vi "PQsyncQueryCommand.vi"(8 "error in (no error)":errorcluster, 9 "query":string, 11 "conn":u64) -> (0 "error out":errorcluster, 1 "PQresultStatus":T1(ring), 2 "PGresult":u64, 3 "conn out":u64, 4 "PQresultErrorMessage":string)   [LabVIEW 2019, in "libpqutility64.lvlib"]
doc: "Synchrounus Communication with PostgreSQL Database.\nSee PostgreSQL c-lib doku for further information."
uses:
  libpqutility64.lvlib
  libpqlv64/libpqlv64.lvlib
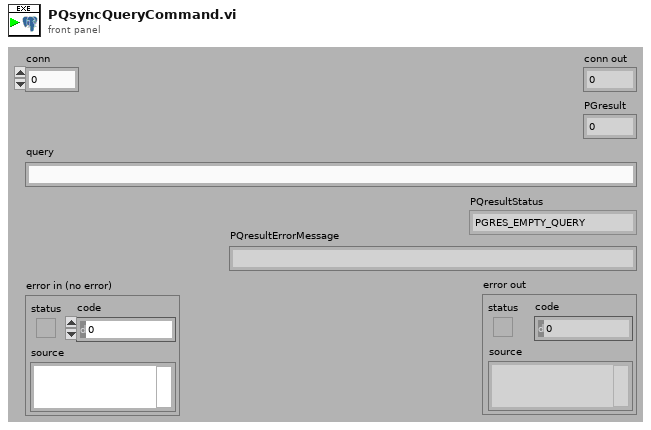
[diagram p1: front panel]
types:
  T1 = enum32{"PGRES_EMPTY_QUERY", "PGRES_COMMAND_OK", "PGRES_TUPLES_OK", "PGRES_COPY_OUT", "PGRES_COPY_IN", "PGRES_BAD_RESPONSE", "PGRES_NONFATAL_ERROR", "PGRES_FATAL_ERROR"}
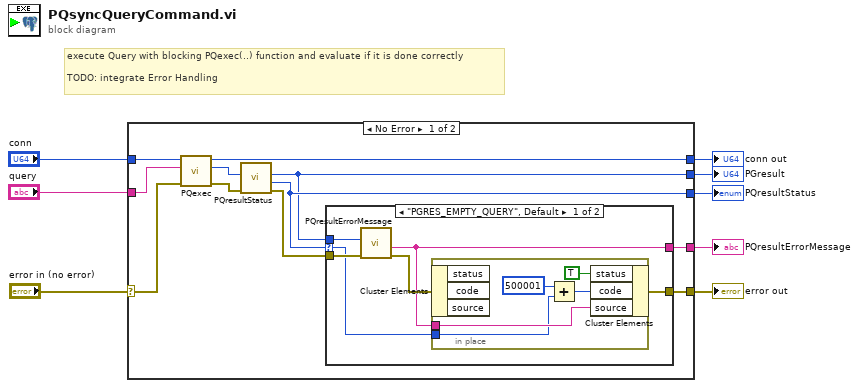
[diagram p0: block diagram]
diagram:
  # "execute Query with blocking PQexec(..) function and evaluate if it is done correctly\n\nTODO: integrate Error Handling"
  n1 = case shown="No Error" "error in (no error)" {
    selector: "error in (no error)" -> [w9 w32]
    tunnel: "query" -> [w19 _]
    tunnel: "conn" -> [w17 w33]
    tunnel: [w14 w32] -> w6
    tunnel: [w13 _] -> w5
    tunnel: [w12 _] -> w4
    tunnel: [w11 w33] -> w3
    tunnel: [w10 _] -> w2
    frame No Error {
      n2 = call "PQexec.vi"("error in (no error)"=w9, "query"=w19, "conn"=w17) -> ("error out"=w16:errorcluster, "PGresult"=w18:u64, "conn out"=w11:u64)  [unwired: 6 in]
      n3 = call "PQresultStatus.vi"("error in (no error)"=w16, "res"=w18) -> ("error out"=w15:errorcluster, "PQresultStatus"=w13:T1, "res out"=w10:u64)  [unwired: 7 in]
      n4 = case shown="\"PGRES_EMPTY_QUERY\", Default" w13 {
        selector: w13 -> [w21 _]
        tunnel: w15 -> [w24 w31]
        tunnel: [w22 w31] -> w14
        tunnel: w10 -> [w25 _]
        tunnel: [w20 _] -> w12
        frame "PGRES_EMPTY_QUERY", Default {
          n5 = call "PQresultErrorMessage.vi"("error in (no error)"=w24, "res"=w25) -> ("error out"=w23:errorcluster, "PQresultErrorMessage"=w20:string)  [unwired: 7 in, 1 out]
          n6 = in-place {
            in-place-border: w20 -> [w30]
            in-place-border: w21 -> [w27]
            n7 = in-place-cluster #1(w23) -> ()  [unwired: 3 out]
            n8 = Add(x=u32 500001, y=w27) -> (x+y=w26:u32)
            n9 = in-place-cluster #1("status"=TRUE, "code"=w26, "source"=w30) -> (w22:errorcluster)
          }
        }
        frame "PGRES_COMMAND_OK" {
        }
      }
    }
    frame Error {
    }
  }
  "PQresultStatus" <- w5
  "PQresultErrorMessage" <- w4
  "PGresult" <- w2
  "conn out" <- w3
  "error out" <- w6
